vi "Comparison.vi"(4 "Comparison parameter":T2, 6 "Muticol listbox IN":string[][](array[string]), 7 "Data Stack IN":refnum<class "Retrieved Data.lvclass">[](array[class])) -> (3 "Comparison out":T1)   [LabVIEW 2017, in "Retrieved Data.lvclass"]
uses:
  Retrieved Data.lvclass
  Comparison OUT.ctl
  Retrieved Data.lvclass/Retrieved Data.ctl
  <vilib>/Analysis/baseanly.llb/Mean (DBL).vi
  <vilib>/Analysis/NI_AALPro.lvlib
  <vilib>/Analysis/NI_AALBase.lvlib
panel:
  out "최소값":dbl
  out "최대값":dbl
  out "Output (flattened)":string="1\t10\t100\n2\t11\t110\n3\t12\t120\n4\t13\t130\n5\t14\t140\n6\t15\t150\n7\t16\t160\n8\t17\t170\n9\t18\t180\n"
  out "Statistics 2":dbl
  out "Statistics":dbl
  in  "p-value":dbl format="%#_13g"
  out "Dmax (Amplitude)":dbl
  out "KS table (Amplitude)":dbl[][](array[numeric])
  out "Dmax (IEI)":dbl
  out "KS table (IEI)":dbl[][](array[numeric])
  out "Mean frequency":cluster{dbl[], dbl[]}[](graph)
  out "Mean amplitude":cluster{dbl[], dbl[]}[](graph)
  out "CP_Amplitude":cluster{"X Values":dbl[], dbl[]}[](graph)
  out "CP_IEI":cluster{"X Values":dbl[], dbl[]}[](graph)
  out "t-Test Statistics":T3(array[cluster])
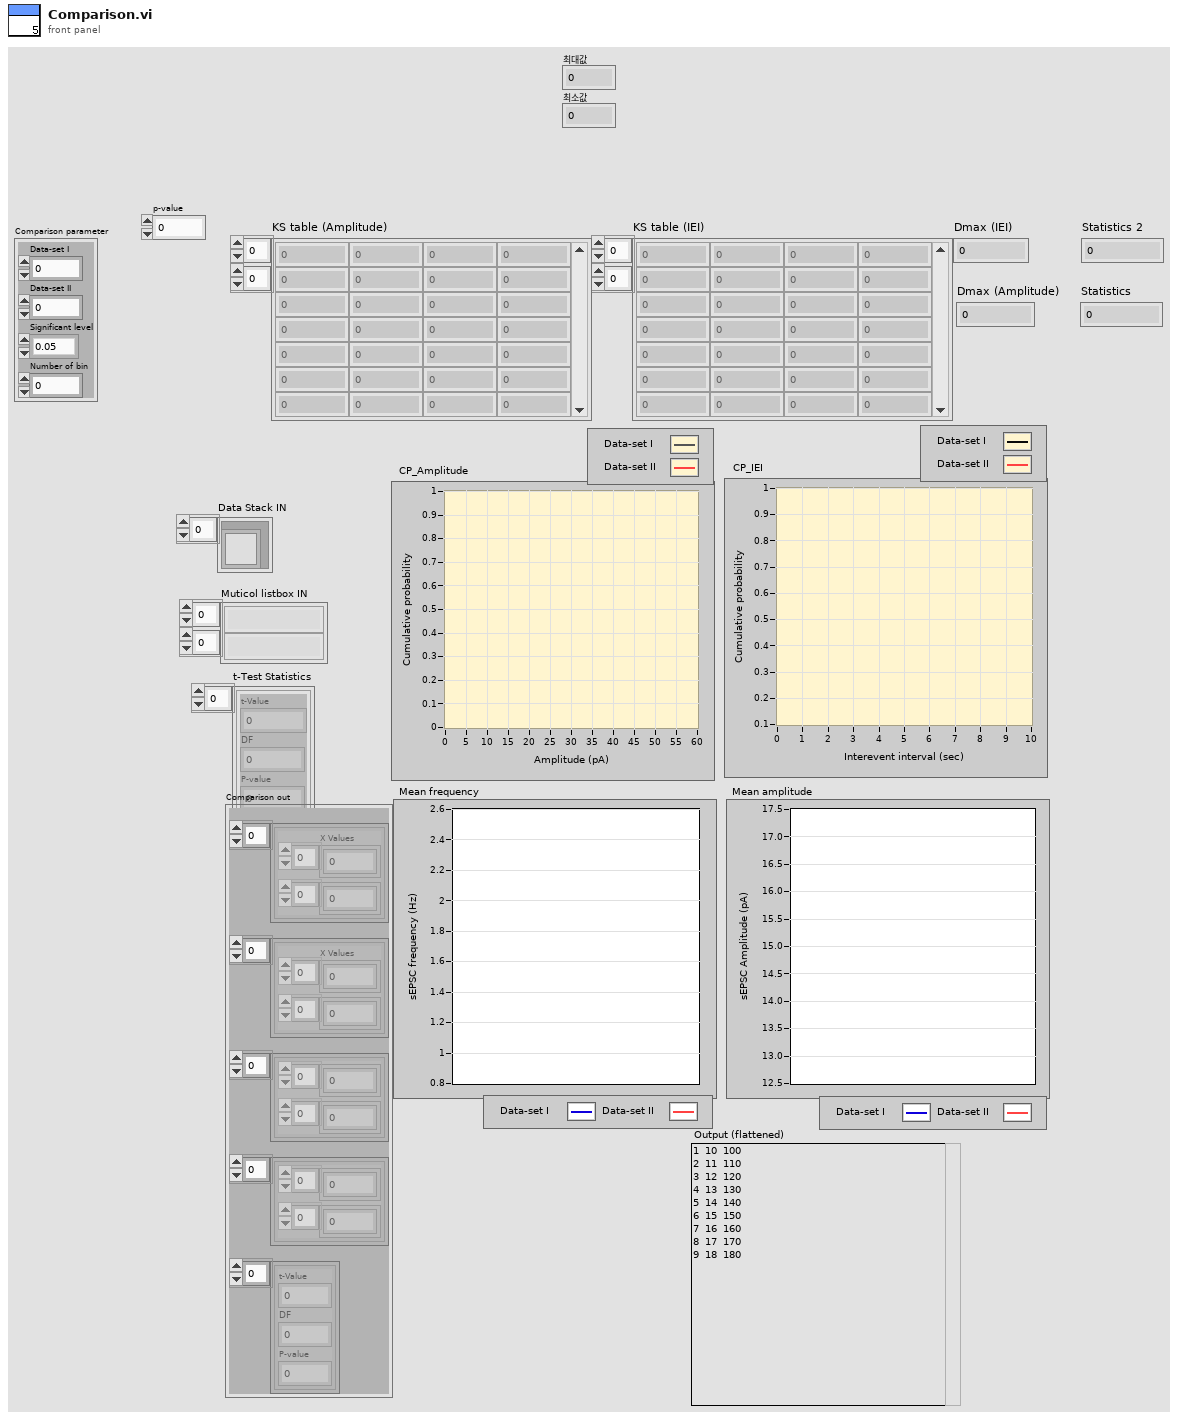
[diagram p1: front panel]
types:
  T1 = typedef "Comparison OUT.ctl" = cluster{"CP_Amplitude":cluster{"X Values":dbl[], dbl[]}[], "CP_IEI":cluster{"X Values":dbl[], dbl[]}[], "Mean Amplitude":cluster{dbl[], dbl[]}[], "Mean frequency":cluster{dbl[], dbl[]}[], "t-statistics":cluster{"t-Value":dbl, "DF":i32, "P-value":dbl}[]}
  T2 = cluster{"Data-set I":u16, "Data-set II":u16, "Significant level":enum16{"0.05", "0.01"}, "Number of bin":dbl}
  T3 = cluster{"t-Value":dbl, "DF":i32, "P-value":dbl}[]
  T4 = cluster{"X Values":dbl[], "Histogram: h(x)":i32[]}
  T5 = cluster{cluster{"X Values":dbl[], dbl[]}[], cluster{"X Values":dbl[], dbl[]}[], cluster{dbl[], dbl[]}[], cluster{dbl[], dbl[]}[], cluster{"t-Value":dbl, "DF":i32, "P-value":dbl}[]}
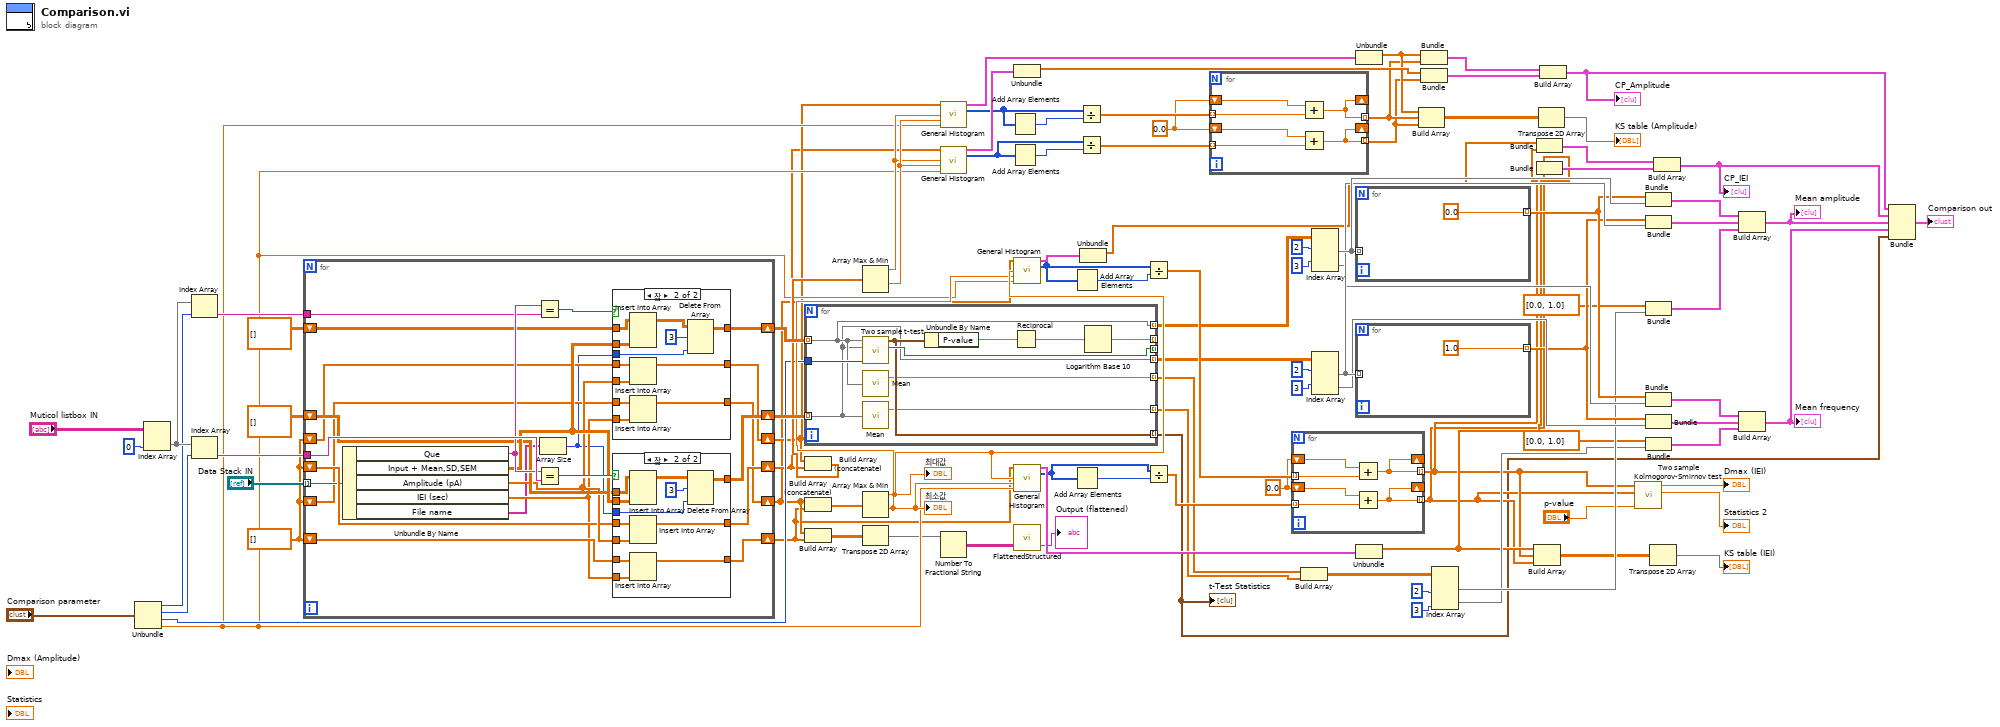
[diagram p0: block diagram]
diagram:
  w63 = 0.0
  w66 = 0.0
  w93 = dbl[] []
  n1 = Unbundle("Comparison parameter") -> ("Data-set I"=w33:u16, "Data-set II"=w32:u16, "Significant level"=w31:enum16{"0.05", "0.01"}, "Number of bin"=w29:dbl)
  n2 = Index Array(array="Muticol listbox IN", index (col)=0 ("비활성화된 인덱스 (열)")) -> (element=w34:string[])  [unwired: 1 in]
  n3 = Index Array(array=w34, index=w33) -> (element=w97:string)
  n4 = Index Array(array=w34, index=w32) -> (element=w98:string)
  n5 = for {
    tunnel: "Data Stack IN" -> [w108] mode=indexing
    tunnel: w98 -> [w123]
    tunnel: w97 -> [w121]
    shift-right: [w117] -> w95
    shift-left: dbl[][] [] -> [w114]
    shift-right: [w116] -> w94
    shift-left: dbl[][] [] -> [w115]
    shift-right: [w112] -> w10
    shift-left: w93 -> [w111]
    shift-right: [w110] -> w9
    shift-left: w93 -> [w109]
    shift-right: [w106] -> w8
    shift-left: w93 -> [w107]
    shift-right: [w104] -> w7
    shift-left: w93 -> [w105]
    n6 = Unbundle By Name(w108) -> ("Que"=w122:string, "Input + Mean,SD,SEM"=w118:dbl[][], "Amplitude (pA)"=w113:dbl[], "IEI (sec)"=w103:dbl[], "File name"=w102:string[])
    n7 = Equal?(x=w122, y=w121) -> (x = y?=w120:bool)
    n8 = Equal?(x=w122, y=w123) -> (x = y?=w119:bool)
    n9 = Array Size(array=w102) -> (size(s)=w101:i32)
    n10 = case shown="참" w120 {
      tunnel: w118 -> [_ w128]
      tunnel: [w126 w136] -> w117
      tunnel: w114 -> [w126 w138]
      tunnel: w113 -> [_ w132]
      tunnel: [w125 w134] -> w112
      tunnel: w111 -> [w125 w133]
      tunnel: w107 -> [w124 w131]
      tunnel: [w124 w130] -> w106
      tunnel: w103 -> [_ w129]
      tunnel: w101 -> [_ w127]
      frame False {
      }
      frame True {
        n11 = Insert Into Array(array=w138, new element=w128) -> (w137:dbl[][])  [unwired: 2 in]
        n12 = Insert Into Array(array=w133, new element=w132) -> (w134:dbl[])  [unwired: 1 in]
        n13 = Insert Into Array(array=w131, new element=w129) -> (w130:dbl[])  [unwired: 1 in]
        n14 = Delete From Array(array=w137, length=3 ("길이"), index (col)=w127) -> (array with subset deleted=w136:dbl[][])  [unwired: 1 in, 1 out]
      }
    }
    n15 = case shown="참" w119 {
      tunnel: w118 -> [_ w153]
      tunnel: [w141 w150] -> w116
      tunnel: w115 -> [w141 w152]
      tunnel: w113 -> [_ w146]
      tunnel: [w140 w148] -> w110
      tunnel: w109 -> [w140 w147]
      tunnel: w105 -> [w139 w145]
      tunnel: [w139 w144] -> w104
      tunnel: w103 -> [_ w143]
      tunnel: w101 -> [_ w142]
      frame False {
      }
      frame True {
        n16 = Insert Into Array(array=w152, new element=w153) -> (w151:dbl[][])  [unwired: 2 in]
        n17 = Insert Into Array(array=w147, new element=w146) -> (w148:dbl[])  [unwired: 1 in]
        n18 = Insert Into Array(array=w145, new element=w143) -> (w144:dbl[])  [unwired: 1 in]
        n19 = Delete From Array(array=w151, length=3 ("길이"), index (col)=w142) -> (array with subset deleted=w150:dbl[][])  [unwired: 1 in, 1 out]
      }
    }
  }
  n20 = for {
    tunnel: w95 -> [w157] mode=indexing
    tunnel: w94 -> [w156] mode=indexing
    tunnel: [w161] -> w2 mode=indexing
    tunnel: w31 -> [w163]
    tunnel: [w162] -> _ mode=indexing
    tunnel: [w158] -> _ mode=indexing
    tunnel: [w157] -> w62 mode=indexing
    tunnel: [w156] -> w58 mode=indexing
    tunnel: [w155] -> w45 mode=indexing
    tunnel: [w154] -> w46 mode=indexing
    n21 = call <userlib>:"Two sample t-test.vi"("Significant level"=w163, "Data SET II"=w156, "Data SET I"=w157) -> ("Reject null hypothesis"=w162:bool, "t-Test Statistics"=w161:cluster{"t-Value":dbl, "DF":i32, "P-value":dbl})  [unwired: 3 in]
    n22 = call-poly <vilib>:"Mean.vi"("X"=w157) -> ("mean"=w155:dbl)  [unwired: 1 out]
    n23 = call-poly <vilib>:"Mean.vi"("X"=w156) -> ("mean"=w154:dbl)  [unwired: 1 out]
    n24 = Unbundle By Name(w161) -> ("P-value"=w159:dbl)
    n25 = Reciprocal(x=w159) -> (1/x=w160:dbl)
    n26 = Logarithm Base 10(1:w160) -> (0:w158:dbl)
  }
  "t-Test Statistics" <- w2
  n27 = Build Array (concatenate)(w10, w9) -> (w90:dbl[])
  n28 = Build Array (concatenate)(w8, w7) -> (w91:dbl[])
  n29 = Build Array(w8, w7) -> (w12:dbl[][])
  n30 = Array Max & Min(array=w90) -> (max value=w79:dbl, min value=w80:dbl)  [unwired: 2 out]
  n31 = Array Max & Min(array=w91) -> (max value=w84:dbl, min value=w83:dbl)  [unwired: 2 out]
  "최대값" <- w84
  "최소값" <- w83
  n32 = Transpose 2D Array(2D array=w12) -> (transposed array=w11:dbl[][])
  n33 = call <vilib>:"General Histogram.vi"("X"=w10, "max"=w79, "min"=w80, "# bins"=w29) -> ("Histogram Graph"=w73:T4, "Histogram"=w72:i32[])  [unwired: 7 in, 3 out]
  n34 = call <vilib>:"General Histogram.vi"("X"=w9, "max"=w79, "min"=w80, "# bins"=w29) -> ("Histogram Graph"=w76:T4, "Histogram"=w75:i32[])  [unwired: 7 in, 3 out]
  n35 = Number To Fractional String(number=w11) -> (F-format string=w14:string[][])  [unwired: 3 in]
  n36 = Add Array Elements(numeric array=w72) -> (sum=w74:i32)
  n37 = Add Array Elements(numeric array=w75) -> (sum=w78:i32)
  n38 = Unbundle(w76) -> ("X Values"=w77:dbl[])  [unwired: 1 out]
  n39 = call <vilib>:"General Histogram.vi"("X"=w8, "max"=w84, "min"=w83, "# bins"=w29) -> ("Histogram Graph"=w88:T4, "Histogram"=w69:i32[])  [unwired: 7 in, 3 out]
  n40 = call <vilib>:"General Histogram.vi"("X"=w7, "max"=w84, "min"=w83, "# bins"=w29) -> ("Histogram Graph"=w87:T4, "Histogram"=w85:i32[])  [unwired: 7 in, 3 out]
  n41 = call <userlib>:"FlattenedStructured.vi"("Input (structured)"=w14) -> ("Output (flattened)"=→"Output (flattened)":string)  [unwired: 1 in, 1 out]
  n42 = Add Array Elements(numeric array=w69) -> (sum=w89:i32)
  n43 = Add Array Elements(numeric array=w85) -> (sum=w86:i32)
  n44 = Divide(x=w72, y=w74) -> (x/y=w65:dbl[])
  n45 = Divide(x=w75, y=w78) -> (x/y=w64:dbl[])
  n46 = Unbundle(w88) -> ("X Values"=w28:dbl[])  [unwired: 1 out]
  n47 = Divide(x=w69, y=w89) -> (x/y=w68:dbl[])
  n48 = Divide(x=w85, y=w86) -> (x/y=w67:dbl[])
  n49 = for {
    tunnel: w65 -> [w168] mode=indexing
    shift-right: [w167] -> _
    shift-left: w63 -> [w169]
    tunnel: [w167] -> w22 mode=indexing
    tunnel: w64 -> [w165] mode=indexing
    shift-right: [w164] -> _
    shift-left: w63 -> [w166]
    tunnel: [w164] -> w21 mode=indexing
    n50 = Add(x=w169, y=w168) -> (x+y=w167:dbl)
    n51 = Add(x=w166, y=w165) -> (x+y=w164:dbl)
  }
  n52 = for {
    tunnel: w68 -> [w174] mode=indexing
    shift-right: [w173] -> _
    shift-left: w66 -> [w175]
    tunnel: [w173] -> w20 mode=indexing
    tunnel: w67 -> [w171] mode=indexing
    shift-right: [w170] -> _
    shift-left: w66 -> [w172]
    tunnel: [w170] -> w19 mode=indexing
    n53 = Add(x=w175, y=w174) -> (x+y=w173:dbl)
    n54 = Add(x=w172, y=w171) -> (x+y=w170:dbl)
  }
  n55 = Build Array(w45, w46) -> (w44:dbl[][])
  n56 = Index Array(array=w62, index (row) #1=2 ("인덱스 (행)"), index (row) #2=3 ("인덱스 (행)")) -> (element #1=w60:dbl[], element #2=w49:dbl[])  [unwired: 2 in]
  n57 = Index Array(array=w58, index (row) #1=2 ("인덱스 (행)"), index (row) #2=3 ("인덱스 (행)")) -> (element #1=w57:dbl[], element #2=w50:dbl[])  [unwired: 2 in]
  n58 = Unbundle(w73) -> ("X Values"=w24:dbl[])  [unwired: 1 out]
  n59 = for {
    tunnel: [0.0] -> w48 mode=indexing
    tunnel: w60 -> [_] mode=indexing
  }
  n60 = for {
    tunnel: [1.0] -> w47 mode=indexing
    tunnel: w57 -> [_] mode=indexing
  }
  n61 = Unbundle(w87) -> ("X Values"=w27:dbl[])  [unwired: 1 out]
  n62 = Build Array(w24, w22, w21) -> (w23:dbl[][])
  n63 = Bundle("X Values"=w24, w22) -> (w71:cluster{"X Values":dbl[], dbl[]})  [unwired: 1 in]
  n64 = Bundle("X Values"=w77, w21) -> (w70:cluster{"X Values":dbl[], dbl[]})  [unwired: 1 in]
  n65 = Index Array(array=w44, index (col) #1=2 ("비활성화된 인덱스 (열)"), index (col) #2=3 ("인덱스 (열)")) -> (element #1=w41:dbl[], element #2=w40:dbl[])  [unwired: 2 in]
  n66 = Build Array(w27, w20, w19) -> (w26:dbl[][])
  n67 = Bundle("X Values"=w28, w20) -> (w82:cluster{"X Values":dbl[], dbl[]})  [unwired: 1 in]
  n68 = Bundle("X Values"=w27, w19) -> (w81:cluster{"X Values":dbl[], dbl[]})  [unwired: 1 in]
  n69 = Transpose 2D Array(2D array=w23) -> (transposed array=→"KS table (Amplitude)":dbl[][])
  n70 = Build Array(w71, w70) -> (w6:cluster{"X Values":dbl[], dbl[]}[])
  "CP_Amplitude" <- w6
  n71 = call <userlib>:"Two sample Kolmogorov-Smirnov test.vi"("p-value"="p-value", "G(x)"=w19, "F(x)"=w20) -> ("Statistics"=→"Statistics 2":dbl, "Dmax"=→"Dmax (IEI)":dbl)  [unwired: 3 in]
  n72 = Bundle(w48, w60) -> (w56:cluster{dbl[], dbl[]})  [unwired: 1 in]
  n73 = Bundle(w47, w57) -> (w55:cluster{dbl[], dbl[]})  [unwired: 1 in]
  n74 = Bundle(dbl[] [0.0, 1.0], w41) -> (w36:cluster{dbl[], dbl[]})  [unwired: 1 in]
  n75 = Bundle(w48, w49) -> (w51:cluster{dbl[], dbl[]})  [unwired: 1 in]
  n76 = Bundle(w47, w50) -> (w52:cluster{dbl[], dbl[]})  [unwired: 1 in]
  n77 = Bundle(dbl[] [0.0, 1.0], w40) -> (w39:cluster{dbl[], dbl[]})  [unwired: 1 in]
  n78 = Transpose 2D Array(2D array=w26) -> (transposed array=→"KS table (IEI)":dbl[][])
  n79 = Build Array(w82, w81) -> (w5:cluster{"X Values":dbl[], dbl[]}[])
  "CP_IEI" <- w5
  n80 = Build Array(w56, w55, w36) -> (w4:cluster{dbl[], dbl[]}[])
  "Mean amplitude" <- w4
  n81 = Build Array(w51, w52, w39) -> (w3:cluster{dbl[], dbl[]}[])
  "Mean frequency" <- w3
  n82 = Bundle(w6, w5, w4, w3, w2) -> (→"Comparison out":T5)  [unwired: 1 in]
